vi "Generate Display DVR.vi"(8 "Error In":errorcluster, 11 "Display In":refnum<class "Display.lvclass">) -> (0 "Error Out":errorcluster, 3 "Display Out":refnum<class "Display.lvclass">)   [LabVIEW 2021, in "Display.lvclass"]
uses:
  Display.lvclass
  Controls/Data.ctl
  Display Utilities/Public/Controls/2D Dimensions.ctl
  Display Element/Display Element.lvclass
  Public/Controls/RGB Gains.ctl
  Public/Controls/FPGA Reference.ctl
  Display.lvclass/Display.ctl
  Display Utilities/Display Utilities.lvlib
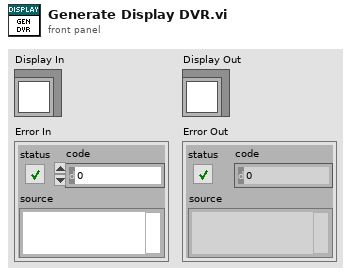
[diagram p1: front panel]
types:
  T1 = typedef "Display.lvclass/Data.ctl" = cluster{"Size":T2, "Display Elements":refnum<class "Display Element.lvclass">[], "Frame":u32[][], "RGB Gains":T3, "FPGA VI Reference":T4}
  T2 = typedef "Display Utilities.lvlib/2D Dimensions.ctl" = cluster{"Width":i32, "Height":i32}
  T3 = typedef "Display.lvclass/RGB Gains.ctl" = cluster{"Red":sgl, "Green":sgl, "Blue":sgl}
  T4 = typedef "Display.lvclass/FPGA Reference.ctl" = refnum<k20>
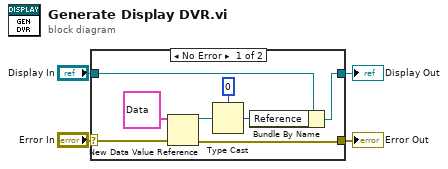
[diagram p0: block diagram]
diagram:
  n1 = case shown="No Error" "Error In" {
    selector: "Error In" -> [w11 w14]
    tunnel: "Display In" -> [w8 w13]
    tunnel: [w5 w14] -> w2
    tunnel: [w6 w13] -> w1
    frame No Error {
      n2 = New Data Value Reference(data value=T1 {"Size"={"Width"=0, "Height"=0}, "Display Elements"=[], "Frame"=[], "RGB Gains"={"Red"=0.0, "Green"=0.0, "Blue"=0.0}, "FPGA VI Reference"=refnum} ("Data"), error in=w11) -> (data value reference=w9:refnum<data-value>, error out=w5:errorcluster)
      n3 = Type Cast(type=u64 0, x=w9) -> (*(type *) &x=w7:u64)
      n4 = Bundle By Name(cluster=w8, "Reference"=w7) -> (w6:refnum<class "Display.lvclass">)
    }
    frame Error {
    }
  }
  "Display Out" <- w1
  "Error Out" <- w2
